vi "Remove String Lines from Multiline String.vi"(2 "Start Index (0)":i32, 3 "Lenght (1)":i32=1, 4 "Multiline String":string) -> (0 "Deleted String":string, 1 "Output String":string)   [LabVIEW 2019]
uses:
  <vilib>/Utility/error.llb/whitespace.ctl
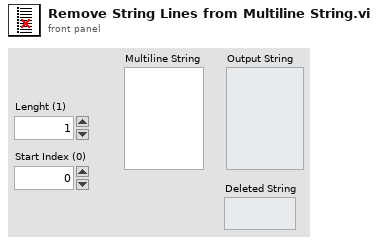
[diagram p1: front panel]
types:
  T1 = typedef "whitespace.ctl" = u16
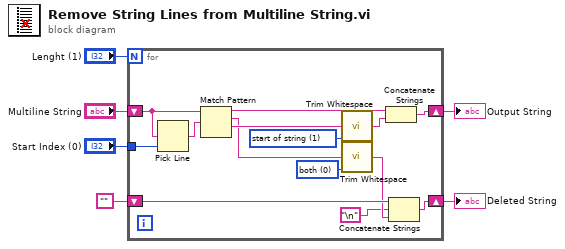
[diagram p0: block diagram]
diagram:
  n1 = for {
    N: "Lenght (1)" -> [_]
    shift-right: [w17] -> w6
    shift-left: "Multiline String" -> [w18]
    tunnel: "Start Index (0)" -> [w20]
    shift-right: [w8] -> w1
    shift-left: "" -> [w10]
    w12 = T1 0 items=["both", "start of string", "end of string"] ("location (both)")
    w14 = T1 1 items=["both", "start of string", "end of string"] ("location (both)")
    n2 = Pick Line(multi-line string=w18, line index=w20) -> (output string=w19:string)  [unwired: 1 in]
    n3 = Match Pattern(string=w18, regular expression=w19) -> (before substring=w13:string, match substring=w11:string, after substring=w16:string)  [unwired: 1 in, 1 out]
    n4 = call <vilib>:"Trim Whitespace.vi"("string"=w16, "location (both)"=w14) -> ("trimmed string"=w15:string)
    n5 = call <vilib>:"Trim Whitespace.vi"("string"=w11, "location (both)"=w12) -> ("trimmed string"=w9:string)
    n6 = Concatenate Strings(w13, w15) -> (w17:string)
    n7 = Concatenate Strings(w10, "\n", w9) -> (w8:string)
  }
  "Output String" <- w6
  "Deleted String" <- w1
